vi "IrDA-Server.vi"() -> ()   [LabVIEW 2019]
doc: "Demonstrates how to set up a basic IrDA connection, send data to the specified service name once a connection has been established, and terminate the connection once the data has been sent. This VI is designed to stop if the IrDA connection is terminated. The data sent in this example is an array of random numbers."
panel:
  in  "Client Closed":string="The client VI closed the connection."
  out "Waveform Graph":dbl[](graph)
  in  "Stop":bool
  # "Overview: Demonstrates the use of the IrDA functions to initialize an IrDA server that can send data to a client VI.\nRequirements: IrDA-enabled computer\nInstructions:\n1. Run the VI.\n2. Open Simple IrDA - Client.vi and follow the instructions on its front panel. Note that if you wait longer than 30 seconds to do this after running this VI, it will time out.\n3. Click Stop to stop the VI. Note that if you stop the client VI, this VI will stop automatically."
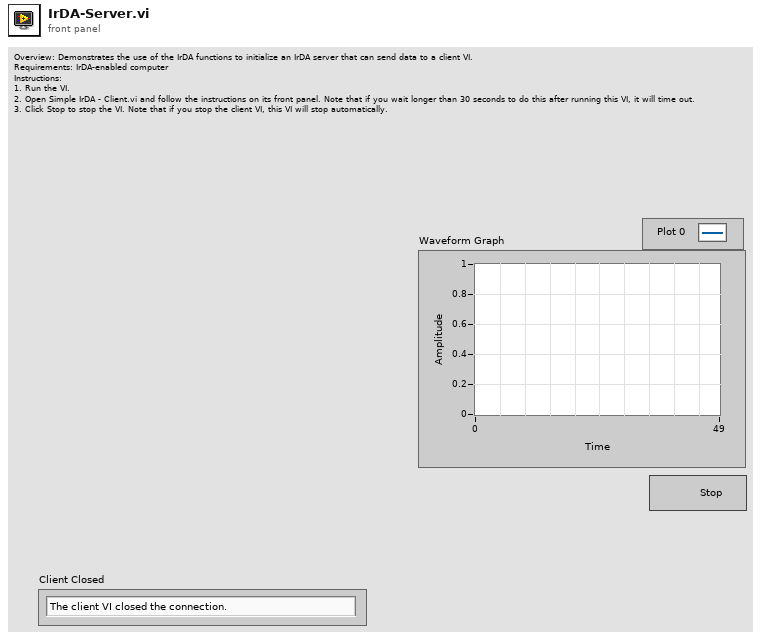
[diagram p1: front panel]
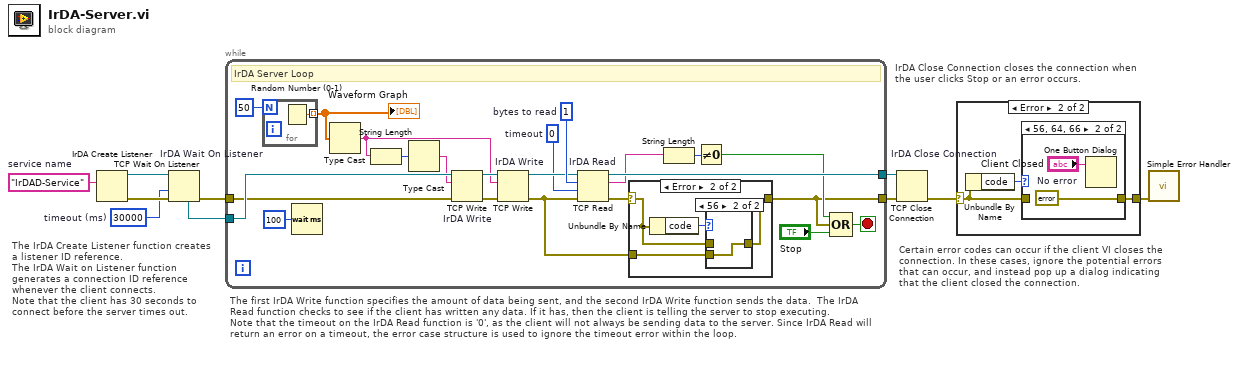
[diagram p0: block diagram]
diagram:
  w2 = "IrDAD-Service"  # service name
  w7 = 30000  # timeout (ms)
  # "IrDA Close Connection closes the connection when the user clicks Stop or an error occurs."
  # "The IrDA Create Listener function creates a listener ID reference. \nThe IrDA Wait on Listener function generates a connection ID reference whenever the client connects. \nNote that the client has 30 seconds to connect before the server times out."
  # "Certain error codes can occur if the client VI closes the connection. In these cases, ignore the potential errors that can occur, and instead pop up a dialog indicating that the client closed the connection."
  # "The first IrDA Write function specifies the amount of data being sent, and the second IrDA Write function sends the data.  The IrDA Read function checks to see if the client has written any data. If it has, then the client is telling the server to stop executing. \nNote that the timeout on the IrDA Read function is '0', as the client will not always be sending data to the server. Since IrDA Read will return an error on a timeout, the error case structure is used to ignore the timeout error within the loop."
  n1 = IrDA Create Listener(10:w2) -> (0:w8:errorcluster, 3:w1:refnum<k19>)  [unwired: 1 in]
  n2 = TCP Wait On Listener "IrDA Wait On Listener"(8:w8, 9:w7, 11:w1) -> (0:w5:errorcluster, 4:w6:refnum<k19>)  [unwired: 1 in, 3 out]
  n3 = while {
    tunnel: [w12] -> w9
    tunnel: [w18] -> w10
    tunnel: w6 -> [w32]
    tunnel: w5 -> [w23]
    stop <- w25 stop-if-true
    w17 = 0  # timeout
    w20 = 1  # bytes to read
    # "IrDA Server Loop"
    n4 = for {
      N: 50 ("# of Points") -> [_]
      tunnel: [w40] -> w21 mode=indexing
      n5 = Random Number (0-1)() -> (number: 0 to 1=w40:dbl)
    }
    "Waveform Graph" <- w21
    n6 = Wait (ms)(milliseconds to wait=u32 100) -> ()  [unwired: 1 out]
    n7 = Type Cast(x=w21) -> (*(type *) &x=w27:string)  [unwired: 1 out]
    n8 = String Length(string=w27) -> (length=w29:i32)
    n9 = Type Cast(x=w29) -> (*(type *) &x=w28:string)  [unwired: 1 out]
    n10 = TCP Write "IrDA Write"(connection ID=w32, data in=w28, error in (no error)=w23) -> (connection ID out=w31:refnum<k19>, error out=w30:errorcluster)  [unwired: 2 out]
    n11 = TCP Write "IrDA Write"(connection ID=w31, data in=w27, error in (no error)=w30) -> (connection ID out=w19:refnum<k19>, error out=w11:errorcluster)  [unwired: 2 out]
    n12 = TCP Read "IrDA Read"(connection ID=w19, bytes to read=w20, error in (no error)=w11, 9:w17) -> (connection ID out=w18:refnum<k19>, data out=w15:string, error out=w13:errorcluster)  [unwired: 1 out]
    n13 = case shown="Error" w13 {
      selector: w13 -> [w33 w36]
      tunnel: [w33 w34] -> w12
      tunnel: w11 -> [_ w35]
      frame No Error {
      }
      frame Error {
        n14 = Unbundle By Name(w36) -> ("code"=w37:i32)
        n15 = case shown="56" w37 {
          tunnel: w36 -> [w38 _]
          tunnel: w35 -> [_ w39]
          tunnel: [w38 w39] -> w34
          frame Default {
          }
          frame 56 {
          }
        }
      }
    }
    n16 = String Length(string=w15) -> (length=w16:i32)
    n17 = Not Equal To 0?(x=w16) -> (x != 0?=w14:bool)
    n18 = Compound Arithmetic op=OR(w14, w12, "Stop") -> (w25:bool)
  }
  n19 = TCP Close Connection "IrDA Close Connection"(connection ID=w10, error in (no error)=w9) -> (error out=w4:errorcluster)  [unwired: 2 out]
  n20 = case shown="Error" w4 {
    selector: w4 -> [w41 w43]
    tunnel: [w41 w42] -> w3
    frame No Error {
    }
    frame Error {
      n21 = Unbundle By Name(w43) -> ("code"=w44:i32)
      n22 = case shown="56, 64, 66" w44 {
        tunnel: w43 -> [w45 _]
        tunnel: [w45 w47] -> w42
        frame Default {
        }
        frame 56, 64, 66 {
          w47 = errorcluster {"status"=FALSE, "code"=0, "source"=""}  # No error
          n23 = One Button Dialog(message="Client Closed") -> ()  [unwired: 1 in, 1 out]
        }
      }
    }
  }
  n24 = call <vilib>:"Simple Error Handler.vi"("error in (no error)"=w3) -> ()  [unwired: 1 in, 8 out]
